vi "write actual configuration.vi"(8 "error in":errorcluster, 10 "Scan Engine configuration in":refnum<class "Scan Engine configuration.lvclass">, 11 "Scan Engine editor node in":refnum<class "Scan Engine editor node.lvclass">) -> (0 "error out":errorcluster, 3 "Scan Engine editor node out":refnum<class "Scan Engine editor node.lvclass">)   [LabVIEW 2013, in "Scan Engine editor node.lvclass"]
uses:
  Scan Engine editor node.lvclass
  <vilib>/NI/TBM Modules/variable/module/configuration/Scan Engine configuration.lvclass
  <vilib>/NI/Tag Bus Data Framework/Configuration Editor/Classes/Module editor node/Write Module Configuration.vi
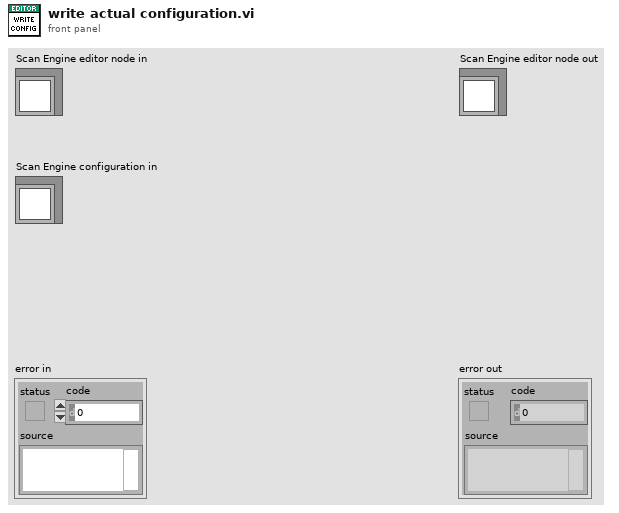
[diagram p1: front panel]
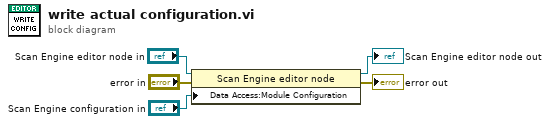
[diagram p0: block diagram]
diagram:
  n1 = property class="Scan Engine editor node"(reference="Scan Engine editor node in", error in="error in", "Data Access:Module Configuration"="Scan Engine configuration in") -> (reference out=→"Scan Engine editor node out":refnum<class "Scan Engine editor node.lvclass">, error out=→"error out":errorcluster)
